vi "Open Shutter.vi"(8 "error in (no error)":errorcluster, 10 "Shutter Enable":bool[](array[boolean])=[FALSE, FALSE, FALSE, FALSE], 11 "Synchronization Device in":refnum<class "Arduino DAQ.lvclass">) -> (0 "error out":errorcluster, 3 "Synchronization Device out":refnum<class "Arduino DAQ.lvclass">)   [LabVIEW 2023, in "Arduino DAQ.lvlib" / "Arduino DAQ.lvclass"]
uses:
  Arduino DAQ.lvclass
  Arduino DAQ.lvclass/Arduino DAQ.ctl
  Arduino DAQ.lvlib
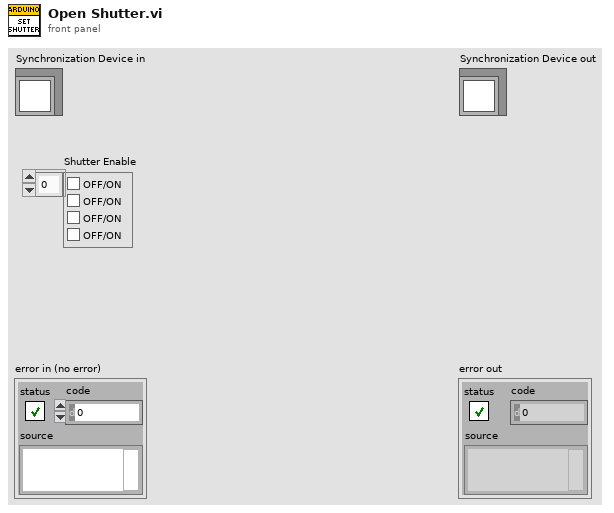
[diagram p1: front panel]
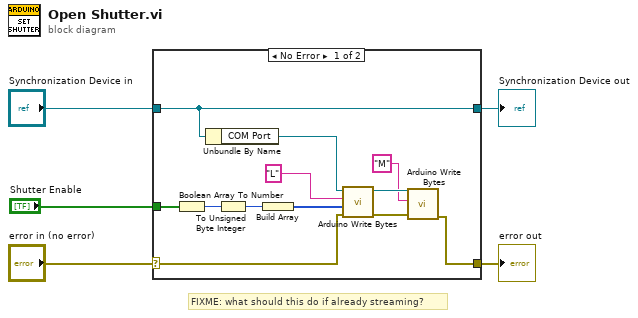
[diagram p0: block diagram]
diagram:
  # "FIXME: what should this do if already streaming?"
  n1 = case shown="No Error" "error in (no error)" {
    selector: "error in (no error)" -> [w16 w19]
    tunnel: [w8 w19] -> w4
    tunnel: [w15 w18] -> w2
    tunnel: "Synchronization Device in" -> [w15 w18]
    tunnel: "Shutter Enable" -> [w17 _]
    frame No Error {
      n2 = Boolean Array To Number(Boolean array=w17) -> (number=w10:u32)
      n3 = Unbundle By Name(w15) -> ("COM Port"=w14:refnum<visa-resource-name>)
      n4 = To Unsigned Byte Integer(number=w10) -> (unsigned 8bit integer=w11:u8)
      n5 = Build Array(w11) -> (w13:u8[])
      n6 = call "Arduino Write Bytes.vi"("error in (no error)"=w16, "Bytes"=w13, "Command"="L", "COM Port In"=w14) -> ("error out"=w9:errorcluster, "COM Port Out"=w7:refnum<visa-resource-name>)  [unwired: 4 in, 2 out]
      n7 = call "Arduino Write Bytes.vi"("error in (no error)"=w9, "Command"="M", "COM Port In"=w7) -> ("error out"=w8:errorcluster)  [unwired: 5 in, 3 out]
    }
    frame Error {
    }
  }
  "error out" <- w4
  "Synchronization Device out" <- w2
